vi "volmetr_auto_filter_freq.vi"(8 "error in (no error)":errorcluster, 10 "measure_freq_value":dbl=160.0, 11 "UI":T1) -> (0 "error out":errorcluster, 3 "output cluster":T1)   [LabVIEW 2017]
uses:
  ui.ctl
  classes/dc_power_supply/DC_power_supply.lvclass
  classes/report/Report.lvclass
  ui_buttons.ctl
  types/boc_type.ctl
  <instrlib>/PICOTEST M352XA/Public/Controls/Function.ctl
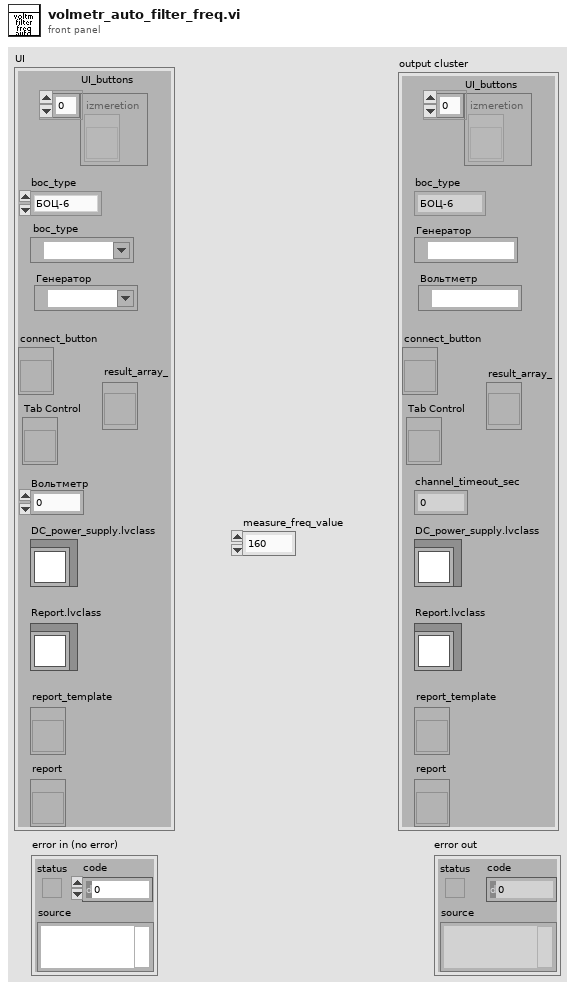
[diagram p1: front panel]
types:
  T1 = typedef "ui.ctl" = cluster{"UI_buttons":T2, "Tab Control":refnum<vi>, "connect_button":refnum<vi>, "generator":refnum<visa-resource-name>, "voltmetr":refnum<visa-resource-name>, "channel_timeout_sec":dbl, "boc_type":T3, "result_array_":refnum<vi>, "DC_power_supply.lvclass":refnum<class "DC_power_supply.lvclass">, "Report.lvclass":refnum<class "Report.lvclass">, "report_template":refnum<vi>, "report":refnum<vi>}
  T2 = typedef "ui_buttons.ctl" = refnum<vi>[]
  T3 = typedef "boc_type.ctl" = enum16{"БОЦ-6", "БОЦ-12"}
  T4 = typedef "Function.ctl" = enum16{"VOLTage:DC", "VOLTage:DC:RATio", "VOLTage:AC", "CURRent:DC", "CURRent:AC", "RESistance", "FRESistance", "FREQuency", "PERiod", "FREQuency:CURRent", "PERiod:CURRent", "CAPacitance", "CONTinuity", "DIODe", "TCOuple", "TEMPerature"}
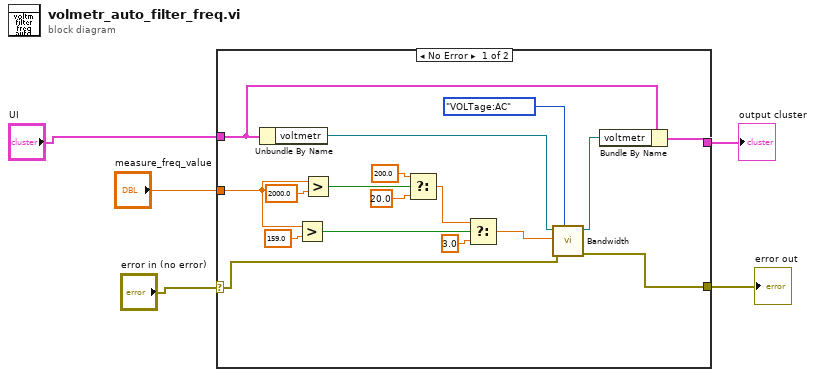
[diagram p0: block diagram]
diagram:
  n1 = case shown="No Error" "error in (no error)" {
    selector: "error in (no error)" -> [w7 w23]
    tunnel: "measure_freq_value" -> [w19 _]
    tunnel: "UI" -> [w11 w24]
    tunnel: [w9 w23] -> w3
    tunnel: [w8 w24] -> w2
    frame No Error {
      n2 = Unbundle By Name(w11) -> ("voltmetr"=w12:refnum<visa-resource-name>)
      n3 = Greater?(x=w19, y=159.0) -> (0:w21:bool)
      n4 = Greater?(x=w19, y=2000.0) -> (0:w17:bool)
      n5 = Select(t=200.0, s=w17, f=20.0) -> (s? t:f=w14:dbl)
      n6 = Select(t=w14, s=w21, f=3.0) -> (s? t:f=w13:dbl)
      n7 = call <instrlib>:"Bandwidth.vi"("Function"=Function."VOLTage:AC", "error in (no error)"=w7, "AC Bandwidth (20: 20 Hz)"=w13, "VISA resource name"=w12) -> ("error out"=w9:errorcluster, "VISA resource name out"=w10:refnum<visa-resource-name>)  [unwired: 5 in, 1 out]
      n8 = Bundle By Name(cluster=w11, "voltmetr"=w10) -> (w8:T1)
    }
    frame Error {
    }
  }
  "error out" <- w3
  "output cluster" <- w2
